vi "2_Anomaly_Threshold(Evaluation).vi"() -> ()   [LabVIEW 2021]
uses:
  Controls/Optimal_Threshold_Range'.ctl
  <vilib>/Ngene/DeepLTK/Toolkit/NN_Network/subVIs/NN_Predict/NN_Predict(In1D_Out1D).vi
  <vilib>/Ngene/DeepLTK/Toolkit/NN_Data/subVIs/Get_Data_Vals/NN_Data_Get_ValByRef(2D_SGL).vi
  <vilib>/Ngene/DeepLTK/Toolkit/Deep_Learning_Toolkit_by_Ngene.lvlib
  <vilib>/Analysis/NI_AALPro.lvlib
panel:
  in  "Validation dataset path":path=path "D:/working/Anomaly Detection/Train"
  in  "Test dataset path":path=path "D:/working/Anomaly Detection/Test"
  out "Integrals of Normalized Anomaly Score Distributions":cluster{"Axis":dbl[], "Integral X":dbl[]}[](graph)
  out "Anomaly Score Distribution":T1(graph)=[{"X Values"=array[700 elements], "Histogram: h(x)"=[0, 0, 0, 0, 0, 0, 0, 0, 0, 0, 0, 0, 0, 0, 0, 0, 0, 0, 0, 0, 0, 0, 0, 0, 0, 0, 0, 0, 0, 0, 0, 0, 0, 0, 0, 0, 1, 2, 5, 5, 8, 9, 5, 13, 9, 12, 13, 17, 13, 20, 12, 18, 18, 17, 20, 14, 17, 15, 19, 8, 9, 11, 14, 16, 9, 10, 16, 7, 6, 10, 10, 6, 9, 4, 4, 8, 3, 1, 5, 3, 2, 3, 5, 5, 3, 2, 3, 2, 2, 1, 4, 3, 0, 2, 0, 1, 1, 2, 3, 0, 1, 0, 0, 0, 0, 0, 0, 0, 0, 1, 0, 1, 1, 0, 0, 0, 0, 0, 0, 0, 1, 0, 0, 0, 0, 0, 0, 0, 0, 0, 0, 0, 0, 0, 0, 0, 0, 0, 0, 0, 0, 0, 0, 0, 0, 0, 0, 0, 0, 0, 0, 0, 0, 0, 0, 0, 0, 0, 0, 0, 0, 0, 0, 0, 0, 0, 0, 0, 0, 0, 0, 0, 0, 0, 0, 0, 0, 0, 0, 0, 0, 0, 0, 0, 0, 0, 0, 0, 0, 0, 0, 0, 0, 0, 0, 0, 0, 0, 0, 0, 0, 0, 0, 0, 0, 0, 0, 0, 0, 0, 0, 0, 0, 0, 0, 0, 0, 0, 0, 0, 0, 0, 0, 0, 0, 0, 0, 0, 0, 0, 0, 0, 0, 0, 0, 0, 0, 0, 0, 0, 0, 0, 0, 0, 0, 0, 0, 0, 0, 0, 0, 0, 0, 0, 0, 0, 0, 0, 0, 0, 0, 0, 0, 0, 0, 0, 0, 0, 0, 0, 0, 0, 0, 0, 0, 0, 0, 0, 0, 0, 0, 0, 0, 0, 0, 0, 0, 0, 0, 0, 0, 0, 0, 0, 0, 0, 0, 0, 0, 0, 0, 0, 0, 0, 0, 0, 0, 0, 0, 0, 0, 0, 0, 0, 0, 0, 0, 0, 0, 0, 0, 0, 0, 0, 0, 0, 0, 0, 0, 0, 0, 0, 0, 0, 0, 0, 0, 0, 0, 0, 0, 0, 0, 0, 0, 0, 0, 0, 0, 0, 0, 0, 0, 0, 0, 0, 0, 0, 0, 0, 0, 0, 0, 0, 0, 0, 0, 0, 0, 0, 0, 0, 0, 0, 0, 0, 0, 0, 0, 0, 0, 0, 0, 0, 0, 0, 0, 0, 0, 0, 0, 0, 0, 0, 0, 0, 0, 0, 0, 0, 0, 0, 0, 0, 0, 0, 0, 0, 0, 0, 0, 0, 0, 0, 0, 0, 0, 0, 0, 0, 0, 0, 0, 0, 0, 0, 0, 0, 0, 0, 0, 0, 0, 0, 0, 0, 0, 0, 0, 0, 0, 0, 0, 0, 0, 0, 0, 0, 0, 0, 0, 0, 0, 0, 0, 0, 0, 0, 0, 0, 0, 0, 0, 0, 0, 0, 0, 0, 0, 0, 0, 0, 0, 0, 0, 0, 0, 0, 0, 0, 0, 0, 0, 0, 0, 0, 0, 0, 0, 0, 0, 0, 0, 0, 0, 0, 0, 0, 0, 0, 0, 0, 0, 0, 0, 0, 0, 0, 0, 0, 0, 0, 0, 0, 0, 0, 0, 0, 0, 0, 0, 0, 0, 0, 0, 0, 0, 0, 0, 0, 0, 0, 0, 0, 0, 0, 0, 0, 0, 0, 0, 0, 0, 0, 0, 0, 0, 0, 0, 0, 0, 0, 0, 0, 0, 0, 0, 0, 0, 0, 0, 0, 0, 0, 0, 0, 0, 0, 0, 0, 0, 0, 0, 0, 0, 0, 0, 0, 0, 0, 0, 0, 0, 0, 0, 0, 0, 0, 0, 0, 0, 0, 0, 0, 0, 0, 0, 0, 0, 0, 0, 0, 0, 0, 0, 0, 0, 0, 0, 0, 0, 0, 0, 0, 0, 0, 0, 0, 0, 0, 0, 0, 0, 0, 0, 0, 0, 0, 0, 0, 0, 0, 0, 0, 0, 0, 0, 0, 0, 0, 0, 0, 0, 0, 0, 0, 0, 0, 0, 0, 0, 0, 0, 0, 0, 0, 0, 0, 0, 0, 0, 0, 0, 0, 0, 0, 0, 0, 0, 0, 0, 0, 0, 0, 0, 0, 0, 0, 0, 0, 0, 0, 0, 0, 0, 0, 0, 0, 0, 0, 0, 0, 0, 0, 0, 0, 0, 0, 0, 0]}, {"X Values"=array[700 elements], "Histogram: h(x)"=[0, 0, 0, 0, 0, 0, 0, 0, 0, 0, 0, 0, 0, 0, 0, 0, 0, 0, 0, 0, 0, 0, 0, 0, 0, 0, 0, 0, 0, 0, 0, 0, 0, 0, 0, 0, 0, 0, 0, 0, 0, 0, 0, 0, 0, 0, 0, 0, 0, 0, 0, 0, 0, 0, 0, 0, 0, 0, 0, 0, 0, 0, 0, 0, 0, 0, 0, 0, 0, 0, 0, 0, 0, 0, 0, 0, 0, 0, 0, 0, 0, 0, 0, 0, 0, 0, 0, 0, 0, 0, 0, 0, 0, 0, 0, 0, 0, 0, 0, 0, 0, 0, 0, 0, 0, 0, 0, 0, 0, 0, 0, 0, 0, 0, 0, 0, 0, 0, 0, 0, 0, 0, 0, 0, 0, 0, 0, 0, 0, 0, 0, 0, 0, 0, 0, 0, 0, 0, 0, 0, 0, 0, 0, 0, 0, 0, 0, 0, 0, 0, 0, 0, 0, 0, 0, 0, 0, 0, 0, 0, 0, 0, 0, 0, 0, 0, 0, 0, 0, 0, 0, 0, 1, 1, 0, 0, 0, 1, 0, 0, 1, 2, 2, 0, 0, 2, 1, 1, 2, 0, 0, 1, 2, 1, 2, 2, 1, 0, 1, 1, 2, 3, 0, 1, 2, 2, 2, 0, 2, 2, 1, 1, 2, 1, 2, 3, 0, 2, 3, 3, 5, 2, 2, 2, 1, 1, 0, 1, 7, 2, 0, 2, 1, 5, 1, 2, 2, 3, 0, 4, 0, 6, 2, 1, 3, 0, 2, 1, 0, 1, 6, 2, 2, 2, 1, 4, 2, 1, 4, 1, 4, 1, 0, 3, 1, 1, 2, 1, 1, 1, 1, 3, 2, 2, 2, 0, 1, 1, 3, 1, 1, 0, 2, 0, 2, 2, 1, 0, 1, 0, 3, 1, 0, 2, 1, 0, 0, 0, 0, 1, 0, 1, 1, 0, 1, 1, 1, 4, 1, 1, 0, 0, 1, 0, 2, 3, 2, 0, 0, 0, 1, 1, 1, 2, 2, 2, 1, 1, 0, 0, 0, 0, 1, 0, 2, 0, 0, 1, 1, 1, 1, 0, 1, 0, 1, 1, 1, 2, 1, 0, 1, 0, 1, 0, 1, 0, 1, 3, 3, 0, 1, 0, 1, 1, 1, 0, 0, 1, 0, 1, 0, 0, 2, 2, 2, 1, 0, 2, 0, 0, 1, 0, 0, 1, 3, 1, 2, 4, 1, 2, 2, 3, 3, 3, 3, 1, 1, 0, 2, 3, 1, 1, 1, 4, 5, 1, 4, 3, 0, 1, 1, 2, 1, 1, 1, 1, 0, 0, 0, 1, 1, 1, 0, 1, 0, 1, 3, 3, 0, 1, 0, 0, 0, 2, 2, 0, 3, 7, 3, 2, 1, 0, 0, 2, 2, 5, 0, 3, 0, 1, 1, 1, 2, 1, 2, 4, 0, 0, 0, 0, 0, 0, 2, 0, 2, 0, 1, 1, 0, 3, 0, 0, 0, 0, 0, 2, 1, 0, 0, 1, 1, 0, 0, 0, 0, 0, 0, 2, 0, 0, 0, 1, 0, 1, 0, 1, 0, 0, 0, 0, 0, 0, 0, 0, 0, 0, 0, 0, 0, 0, 0, 0, 0, 0, 0, 0, 0, 0, 0, 0, 0, 0, 0, 0, 1, 0, 0, 0, 0, 0, 0, 0, 0, 0, 0, 0, 0, 0, 0, 0, 0, 0, 0, 0, 0, 0, 0, 0, 0, 1, 0, 0, 0, 0, 0, 1, 1, 0, 0, 0, 0, 3, 1, 1, 1, 0, 1, 1, 0, 0, 1, 1, 2, 4, 0, 0, 0, 0, 1, 0, 1, 1, 1, 0, 0, 3, 0, 0, 1, 2, 1, 0, 1, 3, 3, 0, 1, 1, 2, 0, 2, 0, 2, 1, 1, 1, 3, 4, 0, 1, 2, 2, 2, 5, 1, 1, 2, 2, 0, 2, 2, 2, 1, 3, 0, 3, 2, 0, 0, 0, 0, 0, 0, 0, 1, 2, 3, 0, 2, 1, 0, 1, 0, 0, 1, 0, 0, 0, 0, 0, 0, 0, 0, 0, 0, 0, 0, 0, 1, 0, 0, 0, 0, 0, 0, 0, 0, 0, 0, 0, 0, 0, 0, 0, 0, 0, 0, 0, 0, 0, 0, 0, 0, 0, 0, 0, 0, 0, 0, 0, 0, 0, 0, 0, 0, 0, 0, 0, 0, 0]}]
  out "Optimal Threshold Range":T2={"Start"=0.17357142857142857, "Stop"=0.245}
  in  "Weights File Path":path=path "D:/Ngene/GitHub/deepltk_examples/2_Waveform_Processing/24_Waveform_Anomaly_Detection/working/Anomaly_Detection/Anomaly_Detection_weights_23_11_21__18_44_57.bin"
  in  "CFG file path":path=path "D:/Ngene/GitHub/deepltk_examples/2_Waveform_Processing/24_Waveform_Anomaly_Detection/working/Anomaly_Detection/Anomaly_Detection_net_cfg_23_11_21__18_44_57.cfg"
  # "Overview: This VI is designed to calculate the optimal anomaly threshold on the generated synthetic dataset.\nRequirements: Deep Learning Toolkit for LabVIEW - https://www.ngene.co/deep-learning-toolkit-for-labview\nInstructions:\n1. Provide \"Network Configuration File Path\" and \"Weight File Path\" generated from \"1_Waveform_Anomaly_Detection(Training).vi\".\n2. Provide Train and Test dataset paths.\n3. Run the VI.\n4.Observe the Range of optimal threshold values.\n5. Choose a value from the range of optimal threshold calculated after the VI stops, and use it as a anomaly detetcion threshold in \"3_Waveform_Anomaly_Detection(Inference).vi\" \n6. Open \"3_Waveform_Anomaly_Detection(Inference).vi\"  to deploy the trained network for inference."
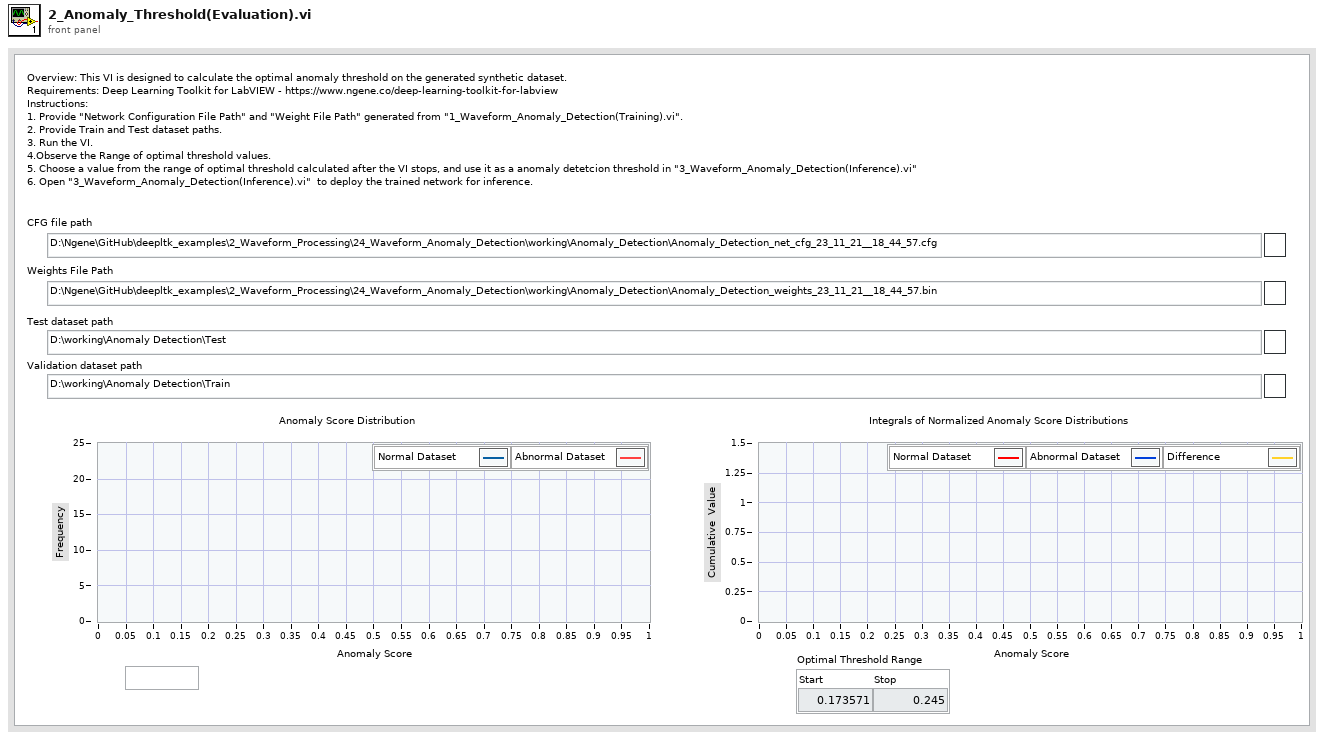
[diagram p1: front panel]
types:
  T1 = cluster{"X Values":dbl[], "Histogram: h(x)":i32[]}[]
  T2 = typedef "Optimal_Threshold_Range'.ctl" = cluster{"Start":dbl, "Stop":dbl}
  T3 = typedef "Deep_Learning_Toolkit_by_Ngene.lvlib/NN_Config_Params.ctl" = cluster{"Name":string, "mBatch":i32, "NN_Train_Params":T4, "LR_Decay_Policy":T7, "Labels":string[], "Loss":T9}
  T4 = typedef "Deep_Learning_Toolkit_by_Ngene.lvlib/NN_Train_Params.ctl" = cluster{"Optimizer":T5, "Beta_1":sgl, "Beta_2":sgl, "Weight Decay(L1)":sgl, "Weight Decay(L2)":sgl, "Data_Sampling":T6}
  T5 = typedef "Deep_Learning_Toolkit_by_Ngene.lvlib/NN_Train_Optimizer.ctl" = enum16{"SGD", "Adam", "Adagrad", "Adadelta", "RMSProp", "Nesterov"}
  T6 = typedef "Deep_Learning_Toolkit_by_Ngene.lvlib/NN_Train_Data_Sampling.ctl" = enum16{"Random", "Sequential"}
  T7 = typedef "Deep_Learning_Toolkit_by_Ngene.lvlib/NN_LR_Policy_Cfg.ctl" = cluster{"Policy_Type":T8, "LR0":dbl, "k":sgl, "WarmUp_Policy":enum16{"Step", "Ramp"}, "WarmUp_Iter":i32, "WarmUp_Ratio":sgl}
  T8 = typedef "Deep_Learning_Toolkit_by_Ngene.lvlib/NN_LR_Policy_Type.ctl" = enum16{"Manual", "Step", "Exp", "1/t"}
  T9 = typedef "Deep_Learning_Toolkit_by_Ngene.lvlib/NN_Loss_Config_Params.ctl" = cluster{"Loss_Type":T10, "Loss_Conf_Params":variant}
  T10 = typedef "Deep_Learning_Toolkit_by_Ngene.lvlib/NN_Loss_Type.ctl" = enum16{"None", "MSE", "CrossEntropy", "YOLO_v2"}
  T11 = typedef "Deep_Learning_Toolkit_by_Ngene.lvlib/NN_Layer_Config_Params.ctl" = cluster{"Layer_Type":T12, "Layer_Conf_Params":variant}
  T12 = typedef "Deep_Learning_Toolkit_by_Ngene.lvlib/NN_Layer_Type.ctl" = enum16{"Input1D", "Input3D", "Conv2D", "Conv2D_Adv", "MaxPool", "AvgPool", "UpSample", "DropOut3D", "ShortCut", "Concat", "SoftMax3D", "FC", "DropOut", "Softmax", "Flatten", "YOLO_v2", "Unsupported"}
  T13 = typedef "Deep_Learning_Toolkit_by_Ngene.lvlib/NN.ctl" = cluster{"Name":string, "No of Layers":i32, "mBatch":i32, "Layers":T14[], "Dimty":T15, "Dims_In":T16, "Dims_Out":T16, "Working_Dir":path, "Train?":bool, "Train_Params":T4, "LR_Update_Policy":T7, "Session Data":T17, "Ground_truth":T18, "NNg_hdls":T20, "NN_Device":T21, "GPU Id":i32, "Labels":string[], "Receptive Field":T22[], "Loss_Type":T10, "Loss_Cfg_Prms":variant}
  T14 = typedef "Deep_Learning_Toolkit_by_Ngene.lvlib/NN_Layer_ref.ctl" = refnum<data-value>
  T15 = typedef "Deep_Learning_Toolkit_by_Ngene.lvlib/NN_In_Out_Dim-ty.ctl" = enum8{"In1D_Out1D", "In3D_Out1D", "In3D_Out3D", "In3D_OutBBox"}
  T16 = typedef "Deep_Learning_Toolkit_by_Ngene.lvlib/NN_Dims(C,H,W).ctl" = cluster{"C":i32, "H":i32, "W":i32}
  T17 = typedef "Deep_Learning_Toolkit_by_Ngene.lvlib/NN_Train_Session_Data.ctl" = cluster{"Epochs":sgl, "Tot_Iter":i32, "LR":sgl, "LR_iter":i32}
  T18 = typedef "Deep_Learning_Toolkit_by_Ngene.lvlib/NN_Ground_truth.ctl" = cluster{"Y":variant, "Y_idx":T19}
  T19 = typedef "Deep_Learning_Toolkit_by_Ngene.lvlib/NN_Data_ref(1D_I32).ctl" = refnum<data-value>
  T20 = typedef "Deep_Learning_Toolkit_by_Ngene.lvlib/nng_cuda_handles.ctl" = cluster{"cudnn":u64, "cublas":u64, "stream":u64, "curand":u64}
  T21 = typedef "Deep_Learning_Toolkit_by_Ngene.lvlib/NN_Device.ctl" = enum16{"CPU", "GPU"}
  T22 = typedef "Deep_Learning_Toolkit_by_Ngene.lvlib/NN_Dims(V,H).ctl" = cluster{"V":i32, "H":i32}
  T23 = typedef "Deep_Learning_Toolkit_by_Ngene.lvlib/NN_DataSets_All(In1D_Out1D).ctl" = cluster{"Train":T24, "Validation":T24, "Test":T24}
  T24 = typedef "Deep_Learning_Toolkit_by_Ngene.lvlib/NN_DataSet(In1D_Out1D).ctl" = cluster{"Inputs Ref.":T25, "Outputs Ref.":T25, "Dims_In":i32, "Dataset_Size":i32, "Outputs_idx Ref.":T19, "Dims_Out":i32, "Labels":string[], "File Paths":path[]}
  T25 = typedef "Deep_Learning_Toolkit_by_Ngene.lvlib/NN_Data_ref(2D_SGL).ctl" = refnum<data-value>
  T26 = cluster{"X Values":dbl[], "Histogram: h(x)":i32[]}
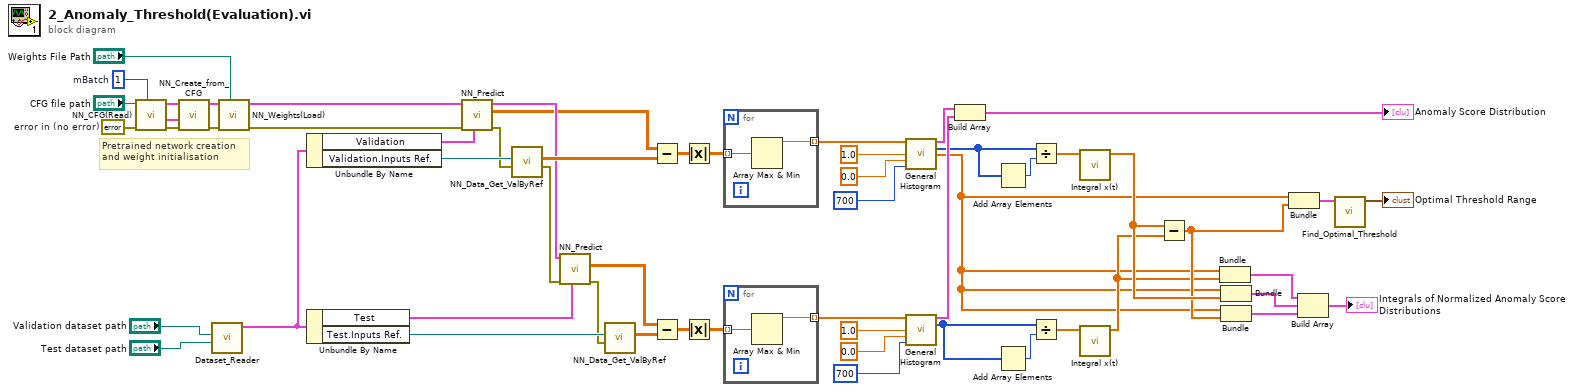
[diagram p0: block diagram]
diagram:
  w51 = 1  # mBatch
  w56 = errorcluster {"status"=FALSE, "code"=0, "source"=""}  # error in (no error)
  # "Pretrained network creation\nand weight initialisation"
  n1 = call <vilib>:"NN_CFG(Read).vi"("mBatch"=w51, "error in (no error)"=w56, "CFG file path"="CFG file path") -> ("error out"=w54:errorcluster, "Net_Cfg"=w55:T3, "Layer_Cfg"=w53:T11[])  [unwired: 6 in]
  n2 = call <vilib>:"NN_Create_from_CFG.vi"("error in (no error)"=w54, "Net_Cfg"=w55, "Layer_Cfg"=w53) -> ("error out"=w57:errorcluster, "NN out"=w52:T13)  [unwired: 7 in]
  n3 = call "Dataset_Reader.vi"("Test dataset path"="Test dataset path", "Validation dataset path"="Validation dataset path") -> ("DataSets_All(In1D_Out1D)"=w5:T23)  [unwired: 8 in, 1 out]
  n4 = call <vilib>:"NN_Weights(Load).vi"("Weight File Path"="Weights File Path", "error in (no error)"=w57, "NN in"=w52) -> ("error out"=w15:errorcluster, "NN out"=w16:T13)  [unwired: 7 in]
  n5 = Unbundle By Name(w5) -> ("Validation"=w48:T24, "Validation.Inputs Ref."=w47:T25)
  n6 = Unbundle By Name(w5) -> ("Test"=w42:T24, "Test.Inputs Ref."=w39:T25)
  n7 = call-poly <vilib>:"NN_Predict.vi"("Dataset"=w48, "error in (no error)"=w15, "NN in"=w16) -> ("error out"=w46:errorcluster, "Predictions"=w35:sgl[][], "NN out"=w41:T13)  [unwired: 6 in]
  n8 = call-poly <vilib>:"NN_Data_Get_ValByRef.vi"("error in (no error)"=w46, "DVR(2D_SGL)"=w47) -> ("error out"=w43:errorcluster, "Value(2D_SGL)"=w45:sgl[][])  [unwired: 6 in]
  n9 = call-poly <vilib>:"NN_Predict.vi"("Dataset"=w42, "error in (no error)"=w43, "NN in"=w41) -> ("error out"=w38:errorcluster, "Predictions"=w36:sgl[][])  [unwired: 6 in, 1 out]
  n10 = call-poly <vilib>:"NN_Data_Get_ValByRef.vi"("error in (no error)"=w38, "DVR(2D_SGL)"=w39) -> ("Value(2D_SGL)"=w37:sgl[][])  [unwired: 6 in, 1 out]
  n11 = Subtract(x=w35, y=w45) -> (x-y=w44:sgl[][])
  n12 = Subtract(x=w36, y=w37) -> (x-y=w40:sgl[][])
  n13 = Absolute Value(x=w44) -> (abs(x)=w34:sgl[][])
  n14 = Absolute Value(x=w40) -> (abs(x)=w33:sgl[][])
  n15 = for {
    tunnel: w34 -> [w59] mode=indexing
    tunnel: [w58] -> w2 mode=indexing
    n16 = Array Max & Min(array=w59) -> (max value=w58:sgl)  [unwired: 3 out]
  }
  n17 = for {
    tunnel: w33 -> [w61] mode=indexing
    tunnel: [w60] -> w3 mode=indexing
    n18 = Array Max & Min(array=w61) -> (max value=w60:sgl)  [unwired: 3 out]
  }
  n19 = call <vilib>:"General Histogram.vi"("X"=w2, "max"=1.0, "min"=0.0, "# bins"=700) -> ("Histogram Graph"=w21:T26, "Histogram"=w19:i32[], "Axis"=w6:dbl[])  [unwired: 7 in, 2 out]
  n20 = call <vilib>:"General Histogram.vi"("X"=w3, "max"=1.0, "min"=0.0, "# bins"=700) -> ("Histogram Graph"=w20:T26, "Histogram"=w24:i32[])  [unwired: 7 in, 3 out]
  n21 = Build Array(w21, w20) -> (→"Anomaly Score Distribution":T1)
  n22 = Add Array Elements(numeric array=w19) -> (sum=w22:i32)
  n23 = Add Array Elements(numeric array=w24) -> (sum=w23:i32)
  n24 = Divide(x=w19, y=w22) -> (x/y=w25:dbl[])
  n25 = Divide(x=w24, y=w23) -> (x/y=w26:dbl[])
  n26 = call <vilib>:"Integral x(t).vi"("X"=w25) -> ("Integral X"=w13:dbl[])  [unwired: 9 in, 1 out]
  n27 = call <vilib>:"Integral x(t).vi"("X"=w26) -> ("Integral X"=w11:dbl[])  [unwired: 9 in, 1 out]
  n28 = Subtract(x=w13, y=w11) -> (x-y=w12:dbl[])
  n29 = Bundle("Axis"=w6, "Integral X"=w11) -> (w10:cluster{"Axis":dbl[], "Integral X":dbl[]})  [unwired: 1 in]
  n30 = Bundle("Axis"=w6, "Integral X"=w13) -> (w9:cluster{"Axis":dbl[], "Integral X":dbl[]})  [unwired: 1 in]
  n31 = Bundle("Axis"=w6, w12) -> (w8:cluster{"Axis":dbl[], dbl[]})  [unwired: 1 in]
  n32 = Bundle("Axis"=w6, w12) -> (w18:cluster{"Axis":dbl[], dbl[]})  [unwired: 1 in]
  n33 = Build Array(w10, w9, w8) -> (→"Integrals of Normalized Anomaly Score Distributions":cluster{"Axis":dbl[], "Integral X":dbl[]}[])
  n34 = call "Find_Optimal_Threshold.vi"("0000000 4"=w18) -> ("Optimal Threshold"=→"Optimal Threshold Range":T2)  [unwired: 10 in]
